vi "Measurement UI.vi"() -> ()   [LabVIEW 2022 SP3, in "Frequency Response UI.lvlib"]
uses:
  Frequency Response UI.lvlib
  shared/controls/sweep profile.ctl
  shared/ui/controls/view.ctl
  shared/controls/input type.ctl
  UI State.ctl
  <vilib>/Utility/miscctls.llb/LVBoundsTypeDef.ctl
  <vilib>/Utility/miscctls.llb/LVPoint32TypeDef.ctl
  <vilib>/Utility/miscctls.llb/LVPointTypeDef.ctl
  Y axis data selection.ctl
  shared/ui/UI Helpers.lvlib
  shared/configuration dialogs/Config Dialog.lvlib
  shared/input configuration file/input cfg file.lvlib
panel:
  in  "view legend":T1
  out "plot point":string
  out "Sweep graph":cluster{"frequency (Hz)":dbl[], "THD+N":dbl[]}[](graph)
  out "Time domain graph":waveform(dbl)[](graph)
  in  "y-axis mapping":enum32{"linear", "logarithmic"}(ring) caption="Y-axis mapping"
  in  "output channel":string="PXI1Slot4/ai0"
  out "ref mic wfm - data":dbl[](array[numeric])
  out "ref mic wfm - dt":dbl
  in  "input cfg file":string
  out "THD":dbl[](array[numeric])
  out "THD+N":dbl[](array[numeric])
  out "amplitude (dBr)":dbl[](array[numeric])
  out "frequency (Hz)":dbl[](array[numeric])
  in  "Configuration tab":T2(tab)
  in  "digital mic sensitivity (dBFS)":dbl=-26.0 caption="Microphone Sensitivity" format="%#.6p dBFS"
  in  "input type":T3 caption="Input Type"
  out "input cfg file name":string
  in  "configure input":bool
  in  "digital channel list":string caption="Digital Audio Channel"
  in  "Output Channel":tag="PXI1Slot2/ao0" caption="Channel"
  in  "Ref Mic Channel":tag="PXI1Slot2/ai0" caption="Channel"
  in  "ref mic sensitivity (mV/Pa)":dbl=50.0 caption="Sensitivity" format="%#.6f mV/Pa"
  in  "output level (dBSPL)":dbl=94.0 caption="Output level" format="%#_3f dBSPL"
  in  "output voltage ratio":dbl=3.39 caption="Output voltage ratio" format="%.3p Pa/V"
  in  "min settling cycles":u32 caption="Minimum settling cycles"
  in  "min settling time (s)":dbl=0.1 caption="Minimum settling time" format="%#_6ps"
  in  "sweep profile":T4=enum."Logarithmic" caption="Profile"
  in  "number of steps":dbl=20000.0 caption="Number of steps"
  in  "start frequency":dbl=20.0 caption="Sweep start" format="%#_6pHz"
  in  "stop frequency":dbl=20000.0 caption="Sweep stop" format="%#_6pHz"
  in  "min measurement cycles":u32 caption="Minimum measurement cycles"
  in  "min measurement time (s)":dbl=0.1 caption="Minimum measurement time" format="%#_6ps"
  in  "x-axis mapping":enum32{"linear", "logarithmic"}(ring) caption="X-axis mapping"
  out "wfm - data":dbl[](array[numeric])
  out "wfm - dt":dbl
  out "channel name":string
  in  "ref mic channel":string="PXI1Slot4/ai0"
  # "hidden controls - used to sync with MeasLink"
  # "hidden for future use"
  # "hidden indicators"
  # "Microphone Interface"
  # "Harware Resource"
  # "Output"
  # "Reference Microphone"
  # "Measurement Settings"
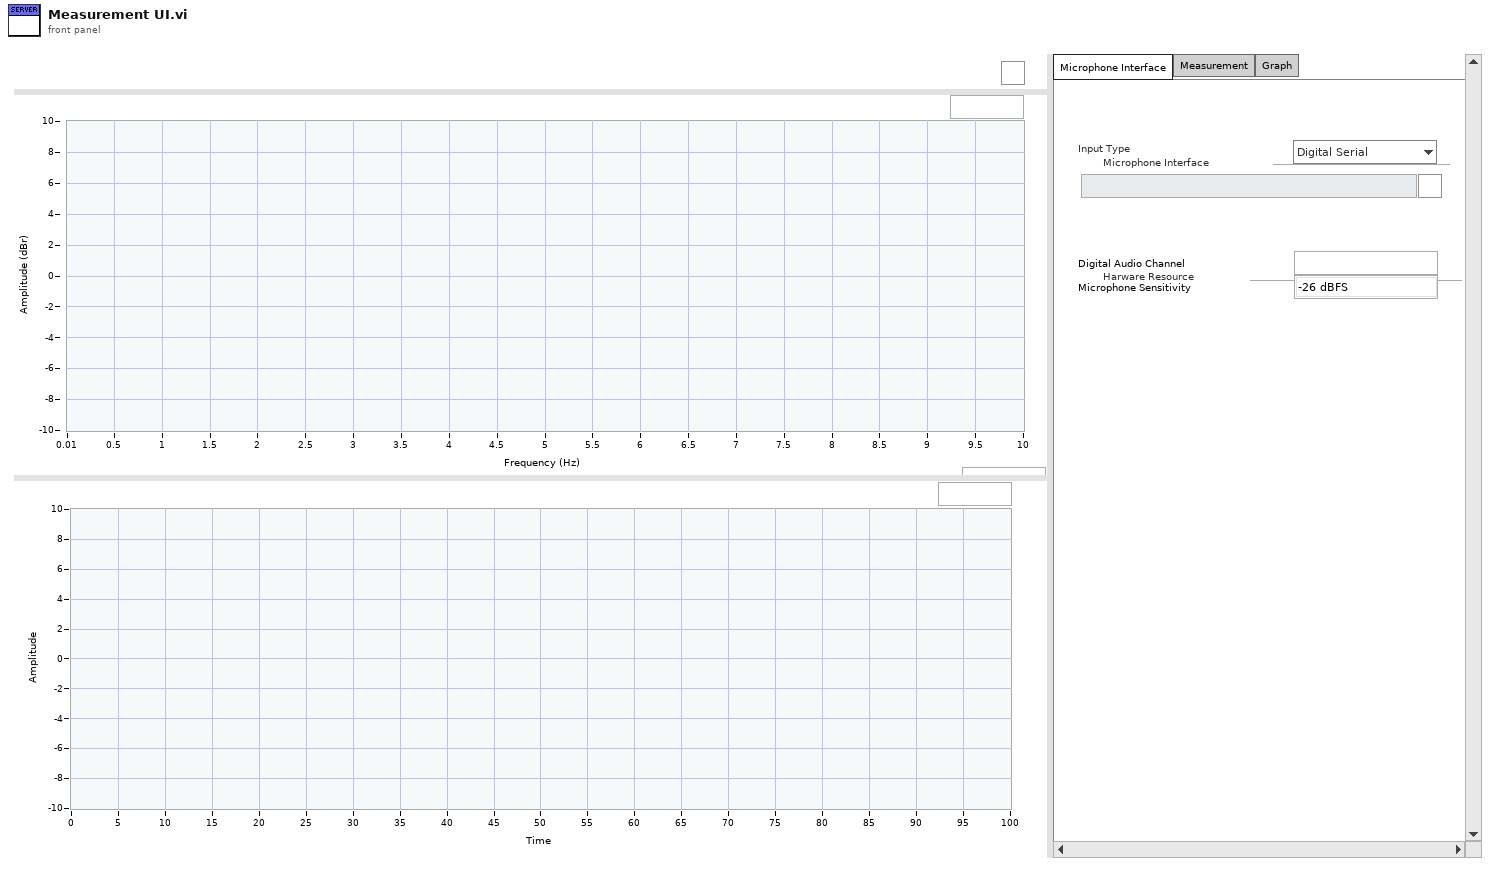
[diagram p1: front panel]
types:
  T1 = typedef "UI Helpers.lvlib/view.ctl" = bool
  T2 = enum32{"Microphone Interface", "Measurement", "Graph"}
  T3 = typedef "input type.ctl" = enum32{"Digital Serial", "PDM"}
  T4 = typedef "sweep profile.ctl" = enum32{"Linear", "Logarithmic"}
  T5 = typedef "Frequency Response UI.lvlib/UI State.ctl" = cluster{"Graph Size":T6, "Legend Visible":bool, "Mouse Coords":T7, "Visible Plot Id":i32, "PostUI event occurred":bool, "input cfg file":path}
  T6 = typedef "LVBoundsTypeDef.ctl" = cluster{"Width":u32, "Height":u32}
  T7 = typedef "LVPoint32TypeDef.ctl" = cluster{"Horizontal":i32, "Vertical":i32}
  T8 = typedef "Frequency Response UI.lvlib/Y axis data selection.ctl" = enum32{"Amplitude (dBr)", "THD (%)", "THD+N (%)"}
  T9 = typedef "LVPointTypeDef.ctl" = cluster{"Horizontal":i16, "Vertical":i16}
  T10 = typedef "Config Dialog.lvlib/audio settings.ctl" = cluster{"input cfg file":string}
  T11 = cluster{"frequency (Hz)":dbl[], "amplitude (dBr)":dbl[]}
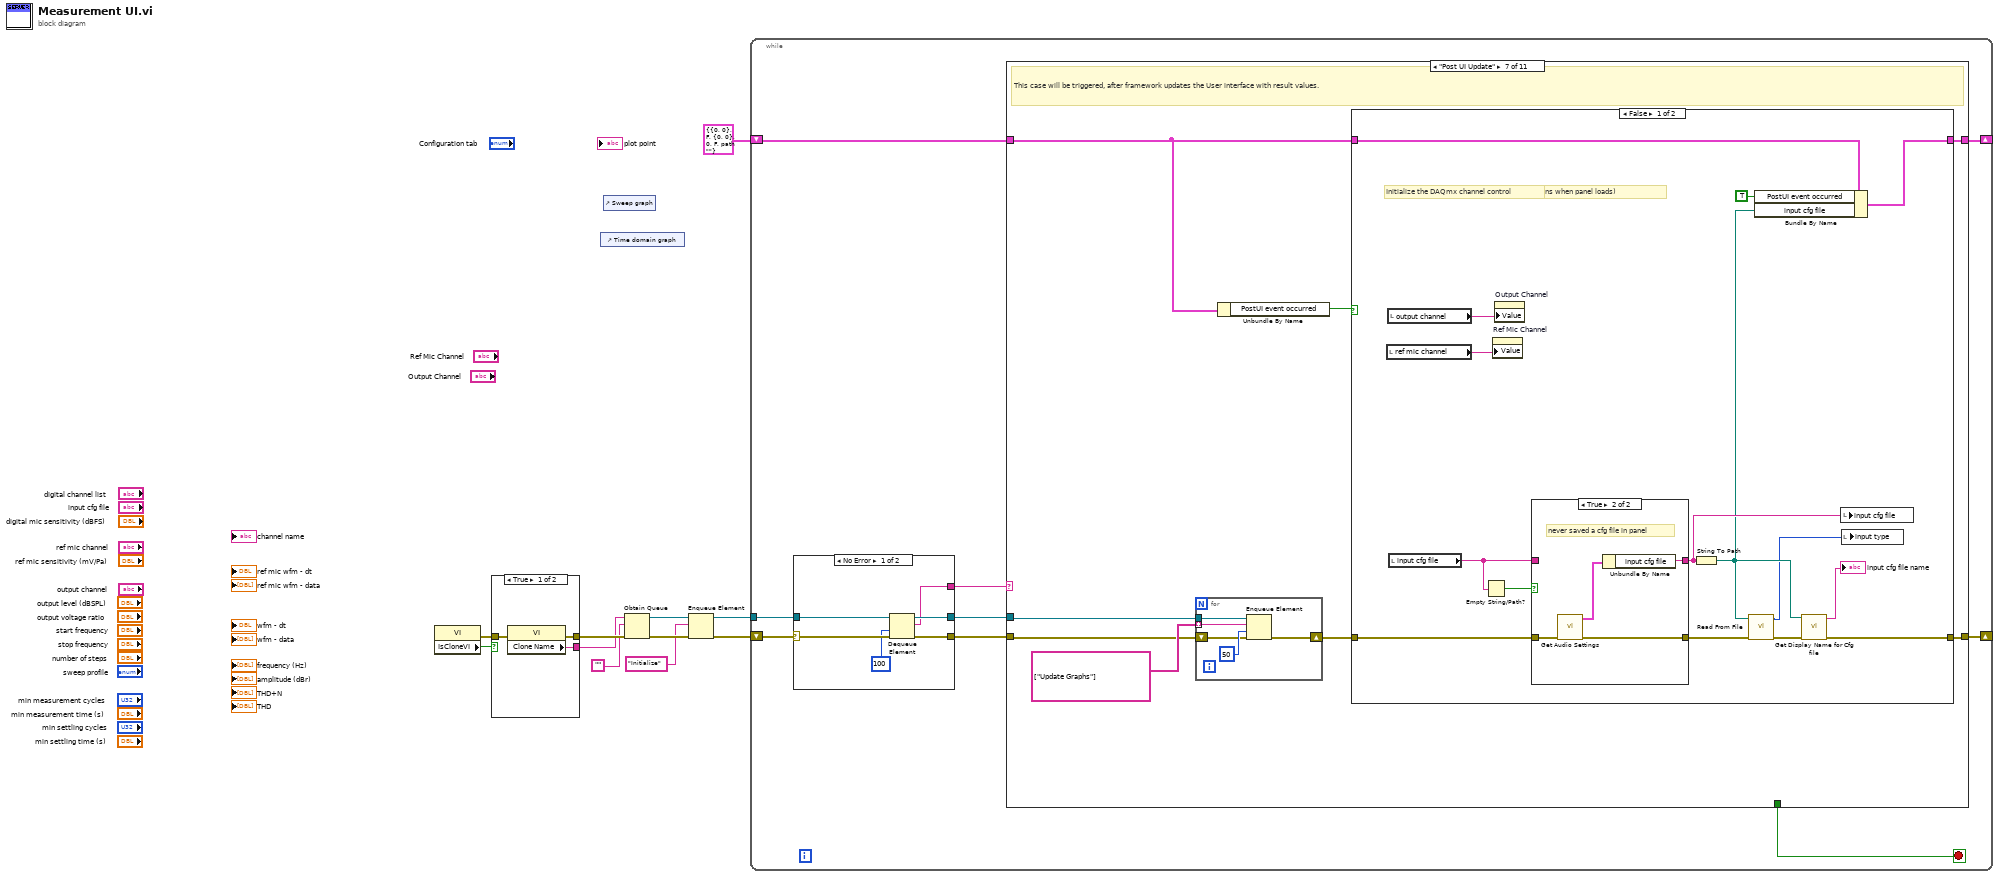
[diagram p0: block diagram]
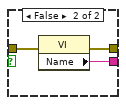
[diagram p2: hidden frame]
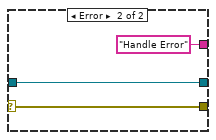
[diagram p3: hidden frame]
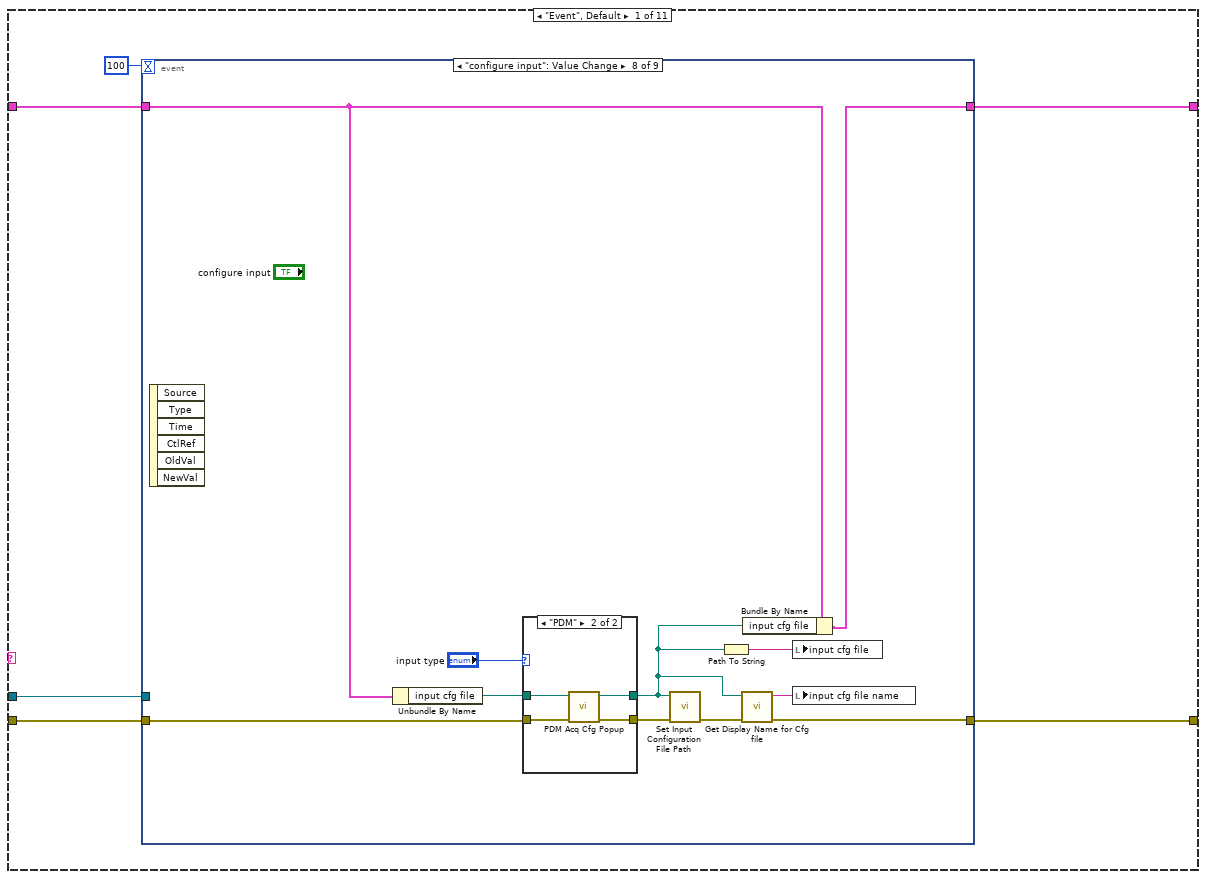
[diagram p4: hidden frame]
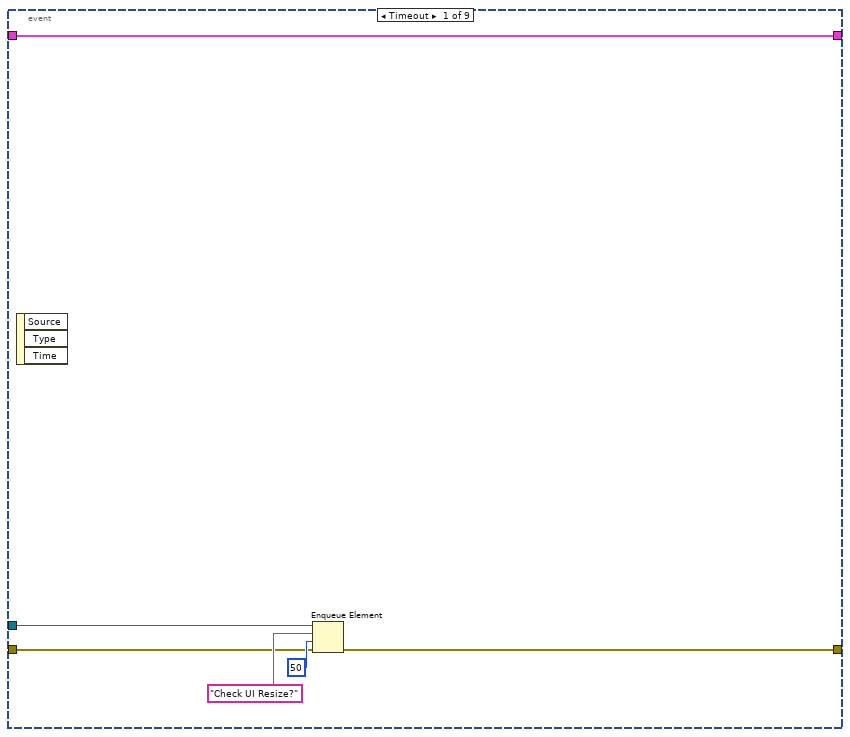
[diagram p5: hidden frame]
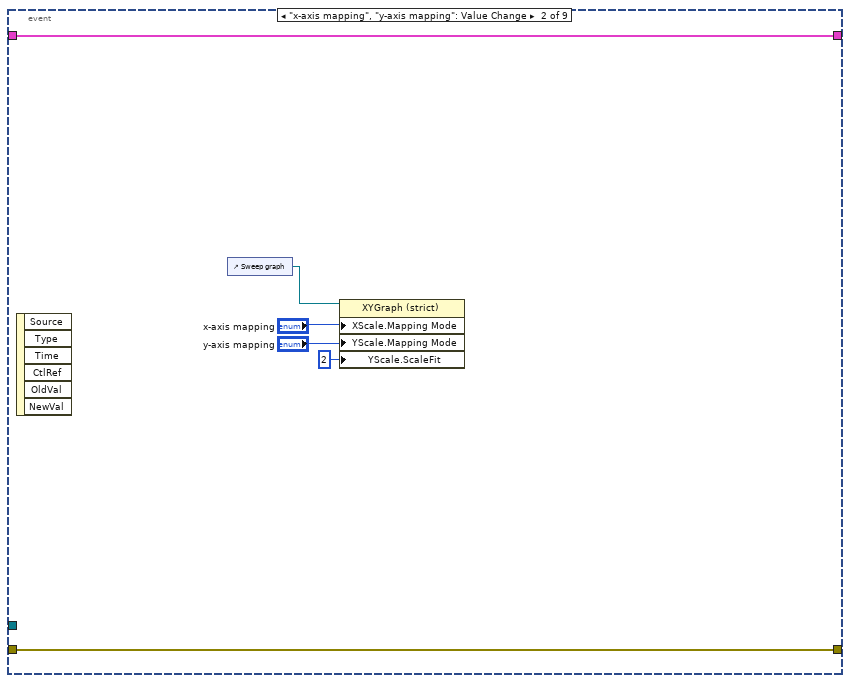
[diagram p6: hidden frame]
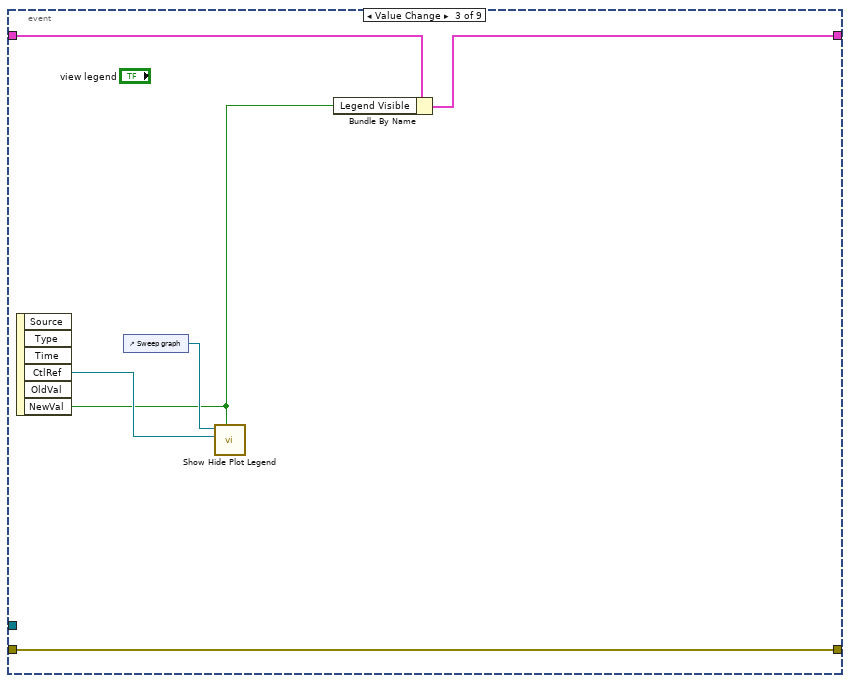
[diagram p7: hidden frame]
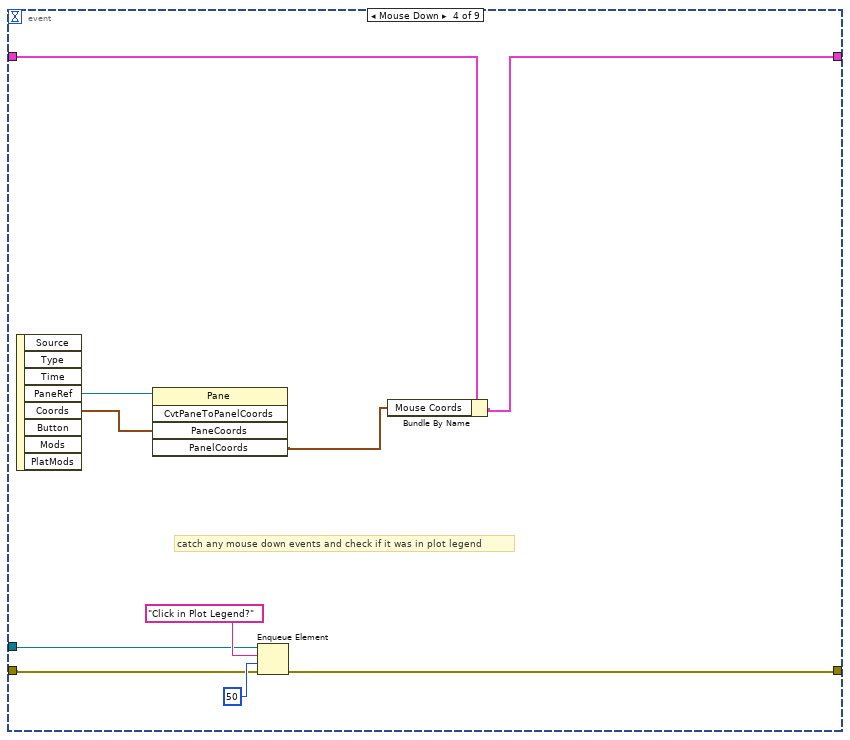
[diagram p8: hidden frame]
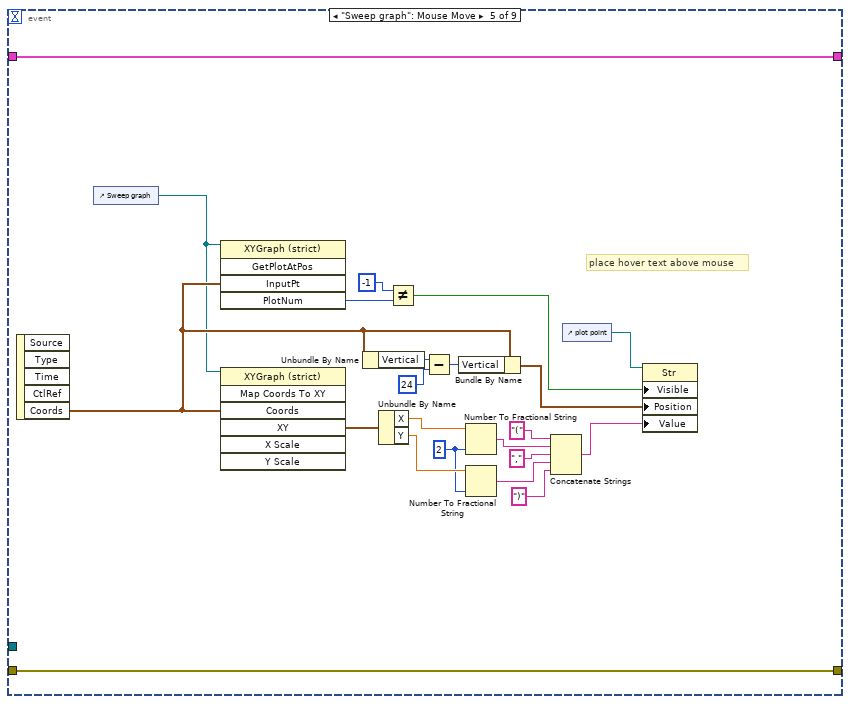
[diagram p9: hidden frame]
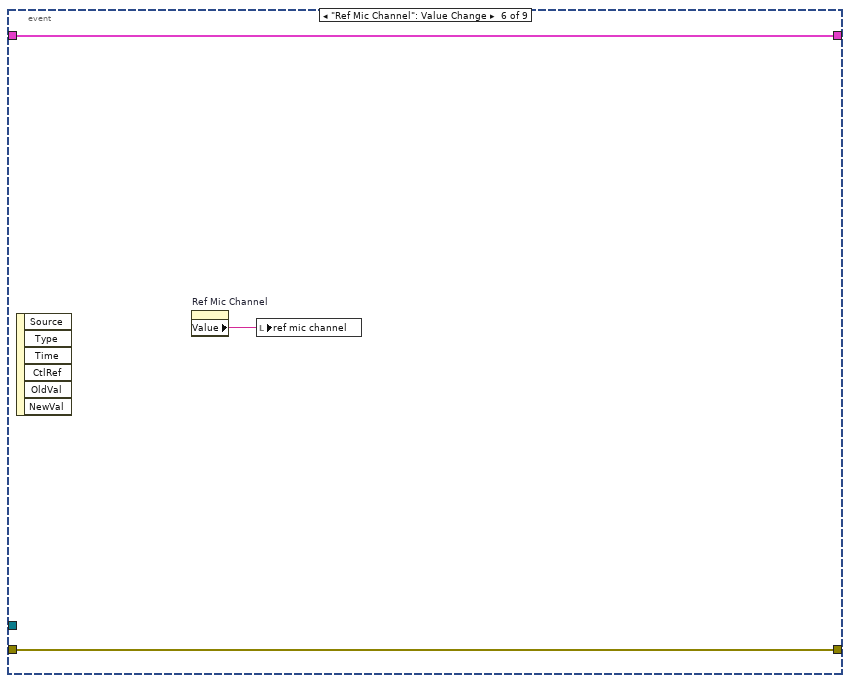
[diagram p10: hidden frame]
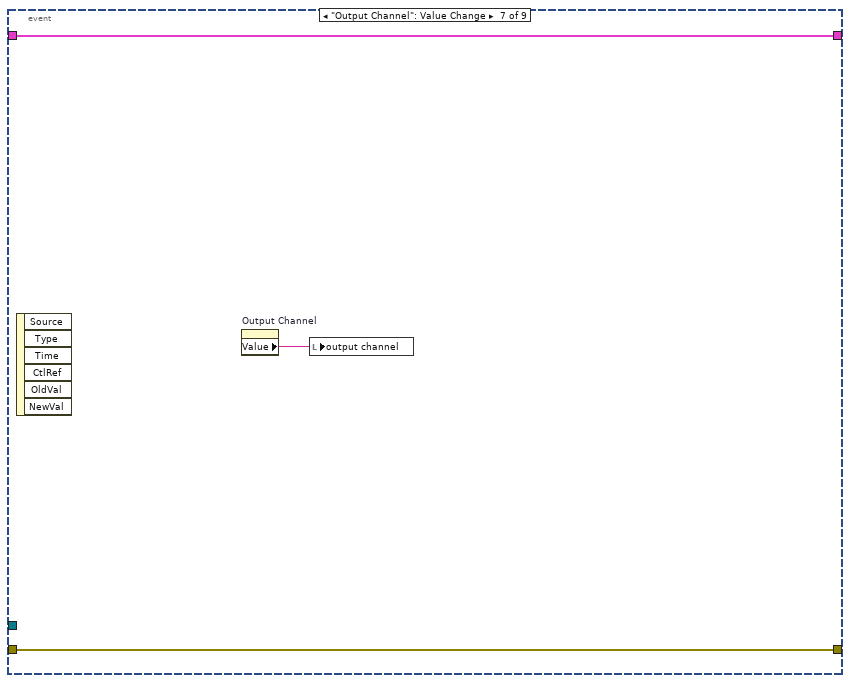
[diagram p11: hidden frame]
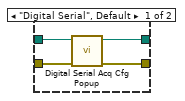
[diagram p12: hidden frame]
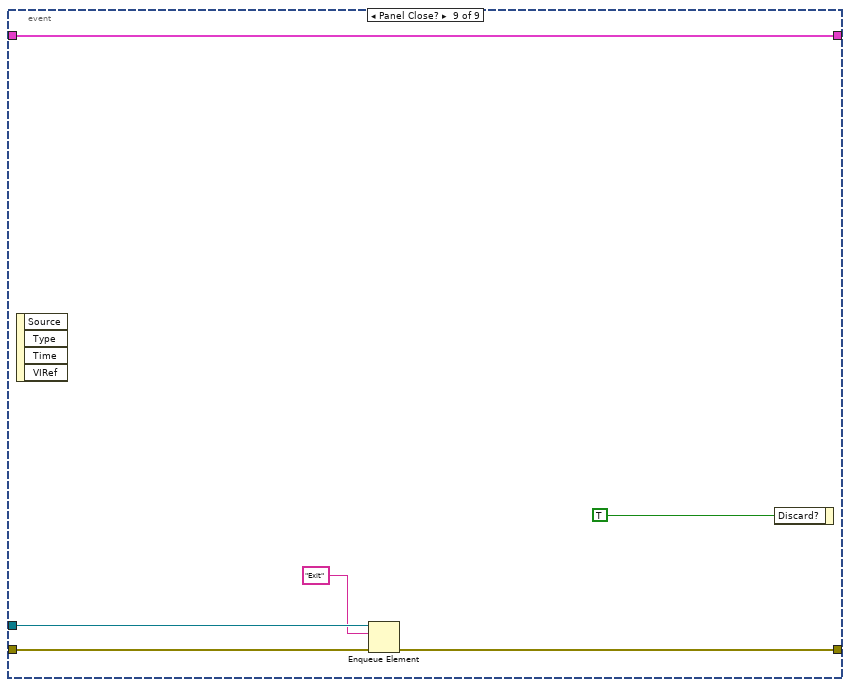
[diagram p13: hidden frame]
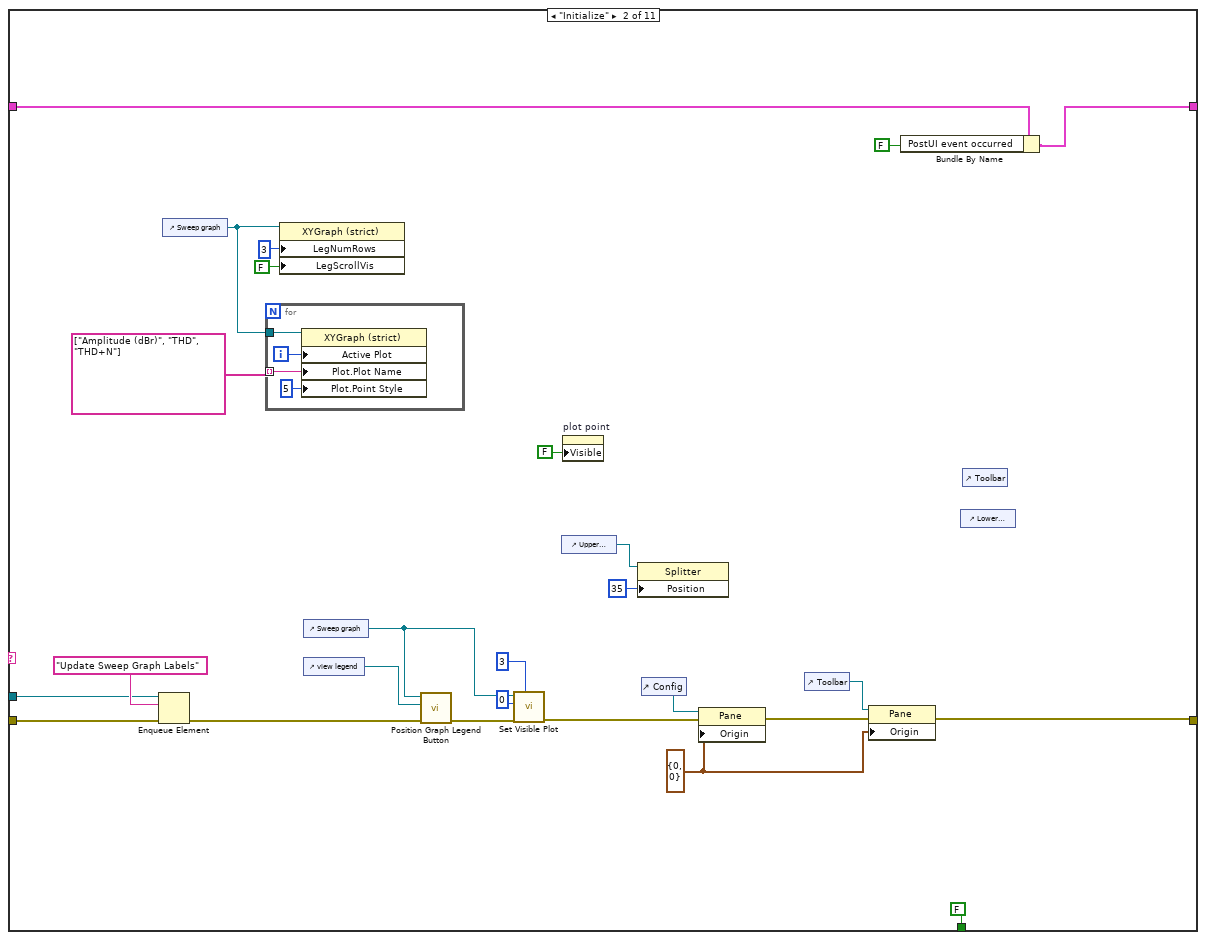
[diagram p14: hidden frame]
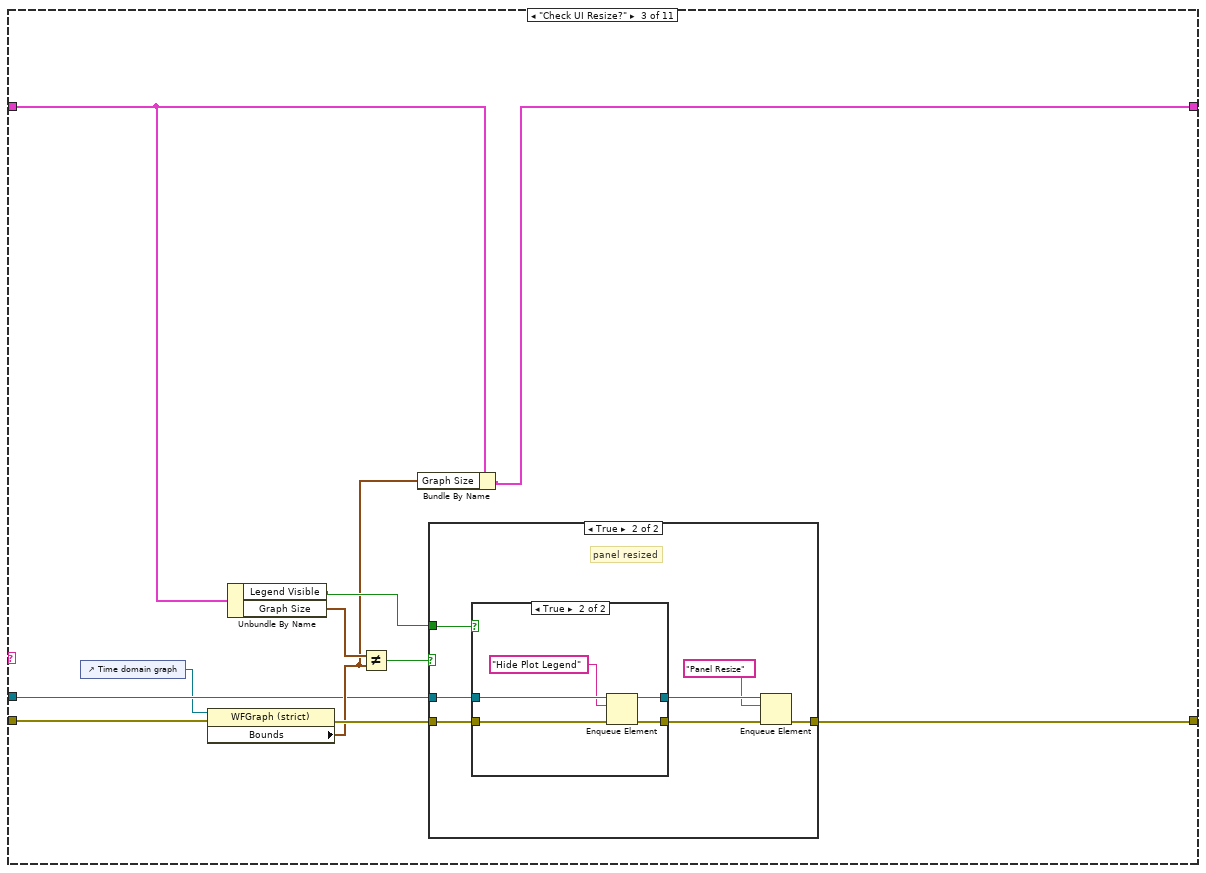
[diagram p15: hidden frame]
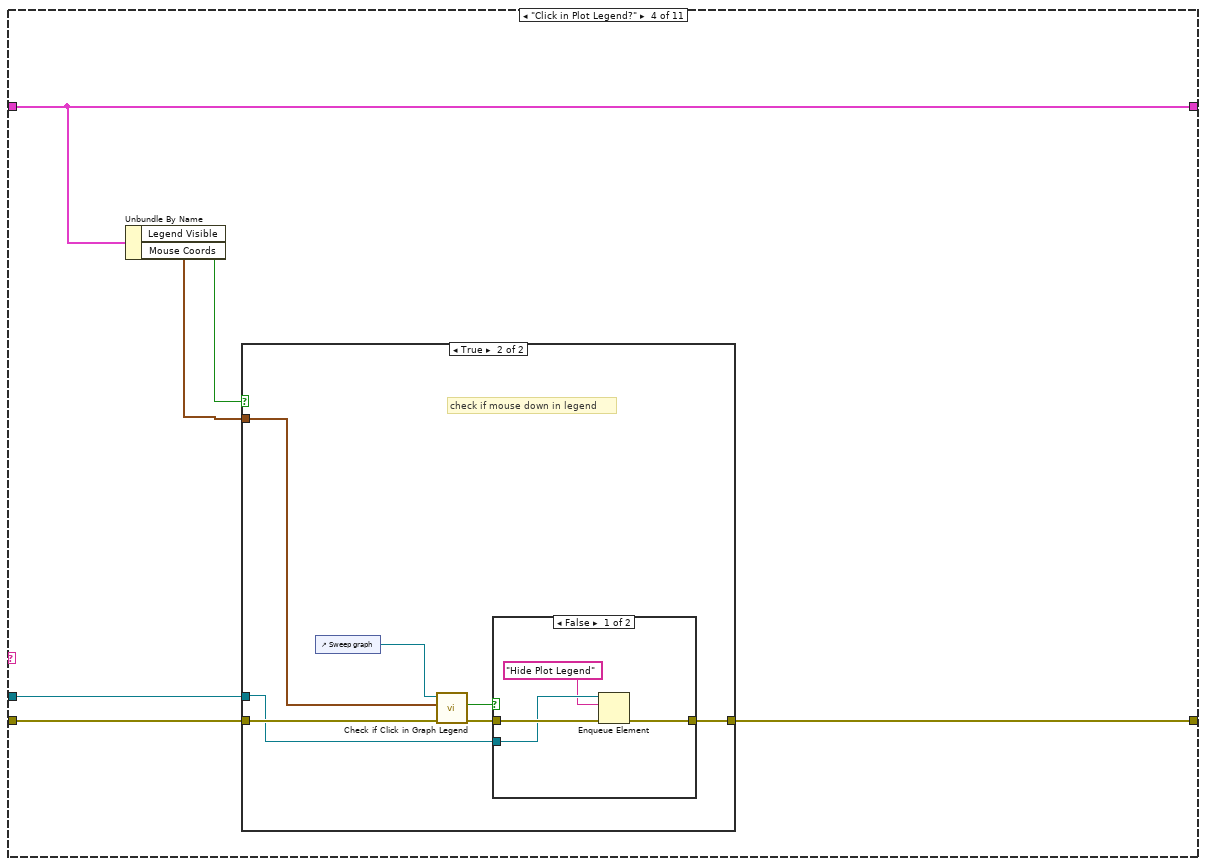
[diagram p18: hidden frame]
diagram:
  n1 = property class="VI"() -> (error out=w2:errorcluster, "IsCloneVI"=w3:bool)  [unwired: 2 in, 1 out]
  n2 = case shown="True" w3 {
    tunnel: [w14 w17] -> w11
    tunnel: [w13 w16] -> w10
    tunnel: w2 -> [w12 w15]
    frame True {
      n3 = property class="VI"(error in=w12) -> (error out=w14:errorcluster, "Clone Name"=w13:string)  [unwired: 1 in, 1 out]
    }
    frame False {
      n4 = property class="VI"(error in=w15) -> (error out=w17:errorcluster, "Name"=w16:string)  [unwired: 1 in, 1 out]
    }
  }
  n5 = control-ref of="Time domain graph"() -> ()  [unwired: 1 out]
  n6 = control-ref of="Sweep graph"() -> ()  [unwired: 1 out]
  n7 = Obtain Queue(name (unnamed)=w10, element data type="", error in (no error)=w11) -> (queue out=w7:refnum<queue>, error out=w9:errorcluster)  [unwired: 2 in, 1 out]
  n8 = Enqueue Element(queue=w7, element="Initialize", error in (no error)=w9) -> (queue out=w6:refnum<queue>, error out=w8:errorcluster)  [unwired: 1 in, 1 out]
  n9 = while {
    shift-right: [w21] -> _
    shift-left: w8 -> [w26]
    tunnel: w6 -> [w24]
    shift-right: [w18] -> _
    shift-left: T5 {"Graph Size"={"Width"=0, "Height"=0}, "Legend Visible"=FALSE, "Mouse Coords"={"Horizontal"=0, "Vertical"=0}, "Visible Plot Id"=0, "PostUI event occurred"=FALSE, "input cfg file"=path ""} ("UI State") -> [w19]
    stop <- w20 stop-if-true
    n10 = case shown="No Error" w26 {
      selector: w26 -> [w32 w35]
      tunnel: [w31 w35] -> w25
      tunnel: w24 -> [w30 w34]
      tunnel: [w29 w34] -> w23
      tunnel: [w28 "Handle Error"] -> w22
      frame No Error {
        n11 = Dequeue Element(queue=w30, timeout in ms (-1)=100, error in (no error)=w32) -> (queue out=w29:refnum<queue>, element=w28:string, error out=w31:errorcluster)  [unwired: 1 out]
      }
      frame Error {
      }
    }
    n12 = case shown="\"Post UI Update\"" w22 {
      tunnel: w25 -> [w40 w139 w157 w182 w202 w207 w216 w262 w271 w279 w281]
      tunnel: w23 -> [w38 w138 w158 w181 _ _ w217 _ _ w277 _]
      tunnel: [w41 w124 w156 w179 w201 w206 w214 w262 w271 w274 w281] -> w21
      tunnel: [_ FALSE _ _ _ _ _ _ _ TRUE _] -> w20
      tunnel: w19 -> [w37 w129 w155 w180 w204 w210 w211 w263 w270 w272 w280]
      tunnel: [w36 w128 w154 w180 w203 w210 w213 w263 w270 w272 w280] -> w18
      frame "Event", Default {
        n13 = event shown="[7] \"configure input\": Value Change" {
          selector: _ -> [_ _ _ _ _ _ _ _ _]
          dyn-events: _ -> [_ _ _ _ _ _ _ _ _]
          timeout: 100 -> [_ _ _ _ _ _ _ _ _]
          tunnel: [w45 w49 w54 w60 w91 w94 w97 w101 w120] -> w41
          tunnel: w40 -> [w44 w49 w54 w61 w91 w94 w97 w102 w121]
          tunnel: w38 -> [w43 _ _ w62 _ _ _ _ w119]
          tunnel: w37 -> [w42 w48 w56 w66 w90 w93 w96 w104 w117]
          tunnel: [w42 w48 w55 w65 w90 w93 w96 w103 w117] -> w36
          event Timeout {
            n14 = event-data() -> ()  [unwired: 1 in, 3 out]
            n15 = Enqueue Element(queue=w43, element="Check UI Resize?", timeout in ms (-1)=50, error in (no error)=w44) -> (error out=w45:errorcluster)  [unwired: 2 out]
          }
          event "x-axis mapping", "y-axis mapping": Value Change {
            n16 = event-data() -> ()  [unwired: 1 in, 6 out]
            n17 = control-ref of="Sweep graph"() -> (w50:refnum<vi>)
            n18 = property on="Property Node" class="XYGraph (strict)"(reference=w50, "XScale.Mapping Mode"="x-axis mapping", "YScale.Mapping Mode"="y-axis mapping", "YScale.ScaleFit"=u8 2 ("Y Scale.Scale Fit")) -> ()  [unwired: 1 in, 2 out]
          }
          event Value Change {
            n19 = event-data() -> ("CtlRef"=w59:refnum<vi>, "NewVal"=w57:T1)  [unwired: 1 in, 4 out]
            n20 = control-ref of="Sweep graph"() -> (w58:refnum<vi>)
            n21 = call "Show Hide Plot Legend.vi"("show"=w57, "view reference"=w59, "graph reference"=w58) -> ()  [unwired: 8 in, 1 out]
            n22 = Bundle By Name(cluster=w56, "Legend Visible"=w57) -> (w55:T5)
          }
          event Mouse Down {
            # "catch any mouse down events and check if it was in plot legend"
            n23 = event-data() -> ("PaneRef"=w68:refnum<vi>, "Coords"=w67:T7)  [unwired: 1 in, 6 out]
            n24 = invoke class="Pane" method="CvtPaneToPanelCoords"(reference=w68, "PaneCoords"=w67) -> ("PanelCoords"=w69:T9)  [unwired: 3 in, 4 out]
            n25 = Enqueue Element(queue=w62, element="Click in Plot Legend?", timeout in ms (-1)=50, error in (no error)=w61) -> (error out=w60:errorcluster)  [unwired: 2 out]
            n26 = Bundle By Name(cluster=w66, "Mouse Coords"=w69) -> (w65:T5)
          }
          event "Sweep graph": Mouse Move {
            w73 = i16 2 ("precision (6)")
            # "place hover text above mouse"
            n27 = event-data() -> ("Coords"=w71:T7)  [unwired: 1 in, 4 out]
            n28 = control-ref of="Sweep graph"() -> (w70:refnum<vi>)
            n29 = invoke class="XYGraph (strict)" method="GetPlotAtPos"(reference=w70, "InputPt"=w71) -> ("PlotNum"=w79:i32)  [unwired: 3 in, 4 out]
            n30 = invoke class="XYGraph (strict)" method="Map Coords To XY"(reference=w70, "Coords"=w71) -> ("XY"=w78:cluster{"X":dbl, "Y":dbl})  [unwired: 5 in, 6 out]
            n31 = Unbundle By Name(w71) -> ("Vertical"=w87:i32)
            n32 = Unbundle By Name(w78) -> ("X"=w84:dbl, "Y"=w85:dbl)
            n33 = Not Equal?(x=-1, y=w79) -> (x != y?=w80:bool)
            n34 = Subtract(x=w87, y=24) -> (x-y=w88:i32)
            n35 = Bundle By Name(cluster=w71, "Vertical"=w88) -> (w86:T7)
            n36 = Number To Fractional String(number=w84, precision (6)=w73) -> (F-format string=w81:string)  [unwired: 2 in]
            n37 = Number To Fractional String(number=w85, precision (6)=w73) -> (F-format string=w82:string)  [unwired: 2 in]
            n38 = Concatenate Strings("(" ("string"), w81, "," ("string"), w82, ")" ("string")) -> (w83:string)
            n39 = control-ref of="plot point"() -> (w89:refnum<vi>)
            n40 = property on="Property Node" class="Str"(reference=w89, "Visible"=w80, "Position"=w86, "Value"=w83) -> ()  [unwired: 1 in, 2 out]
          }
          event "Ref Mic Channel": Value Change {
            n41 = event-data() -> ()  [unwired: 1 in, 6 out]
            n42 = property on="Ref Mic Channel" class="DAQmxName"() -> ("Value"=w92:string)  [unwired: 2 in, 2 out]
            n43 = local write "ref mic channel"(w92) -> ()
          }
          event "Output Channel": Value Change {
            n44 = event-data() -> ()  [unwired: 1 in, 6 out]
            n45 = property on="Output Channel" class="DAQmxName"() -> ("Value"=w95:string)  [unwired: 2 in, 2 out]
            n46 = local write "output channel"(w95) -> ()
          }
          event "configure input": Value Change {
            n47 = event-data() -> ()  [unwired: 1 in, 6 out]
            n48 = Unbundle By Name(w104) -> ("input cfg file"=w108:path)
            n49 = case shown="\"PDM\"" "input type" {
              tunnel: w108 -> [w112 w116]
              tunnel: w102 -> [w111 w115]
              tunnel: [w110 w113] -> w107
              tunnel: [w109 w114] -> w105
              frame "Digital Serial", Default {
                n50 = call "Digital Serial Acq Cfg Popup.vi"("error in (no error)"=w111, "config file in"=w112) -> ("error out"=w110:errorcluster, "config file out"=w109:path)  [unwired: 7 in, 1 out]
              }
              frame "PDM" {
                n51 = call "PDM Acq Cfg Popup.vi"("error in (no error)"=w115, "config file in"=w116) -> ("error out"=w113:errorcluster, "config file out"=w114:path)  [unwired: 7 in, 1 out]
              }
            }
            n52 = call "Set Input Configuration File Path.vi"("error in (no error)"=w107, "configuration file"=w105) -> ("error out"=w106:errorcluster)  [unwired: 9 in]
            n53 = Path To String(path=w105) -> (string=w99:string)
            n54 = call "Get Display Name for Cfg file.vi"("error in (no error)"=w106, "file path"=w105) -> ("error out"=w101:errorcluster, "display string"=w98:string)  [unwired: 8 in]
            n55 = Bundle By Name(cluster=w104, "input cfg file"=w105) -> (w103:T5)
            n56 = local write "input cfg file"(w99) -> ()
            n57 = local write "input cfg file name"(w98) -> ()
          }
          event Panel Close? {
            n58 = event-data() -> ()  [unwired: 1 in, 4 out]
            n59 = Enqueue Element(queue=w119, element="Exit", error in (no error)=w121) -> (error out=w120:errorcluster)  [unwired: 1 in, 2 out]
            n60 = event-data("Discard?"=TRUE) -> ()  [unwired: 1 in, 1 out]
          }
        }
      }
      frame "Initialize" {
        w125 = T9 {"Horizontal"=0, "Vertical"=0} ("Origin")
        n61 = Enqueue Element(queue=w138, element="Update Sweep Graph Labels", error in (no error)=w139) -> (error out=w136:errorcluster)  [unwired: 1 in, 2 out]
        n62 = control-ref of="Sweep graph"() -> (w141:refnum<vi>)
        n63 = for {
          tunnel: string[] ["Amplitude (dBr)", "THD", "THD+N"] -> [w151] mode=indexing
          tunnel: w141 -> [w150]
          i -> [w152]
          n64 = property on="Property Node" class="XYGraph (strict)"(reference=w150, "Active Plot"=w152, "Plot.Plot Name"=w151, "Plot.Point Style"=u8 5) -> ()  [unwired: 1 in, 2 out]
        }
        n65 = property class="XYGraph (strict)"(reference=w141, "LegNumRows"=u32 3 ("Legend:Number of Rows"), "LegScrollVis"=FALSE ("Legend:Scrollbar Visible")) -> ()  [unwired: 1 in, 2 out]
        n66 = control-ref of="Sweep graph"() -> (w135:refnum<vi>)
        n67 = control-ref of="view legend"() -> (w137:refnum<vi>)
        n68 = call "Position Graph Legend Button.vi"("error in (no error)"=w136, "view legend"=w137, "graph"=w135) -> ("error out"=w133:errorcluster)  [unwired: 8 in]
        n69 = call "Set Visible Plot.vi"("number of plots"=3, "error in (no error)"=w133, "Plot Id"=0, "XYGraph in"=w135) -> ("error out"=w132:errorcluster)  [unwired: 7 in]
        n70 = control-ref of="Upper Splitter"() -> (w146:refnum<vi>)
        n71 = property on="plot point" class="Str"("Visible"=FALSE) -> ()  [unwired: 2 in, 2 out]
        n72 = property class="Splitter"(reference=w146, "Position"=35 ("Position:Top")) -> ()  [unwired: 1 in, 2 out]
        n73 = control-ref of="Config"() -> (w147:refnum<vi>)
        n74 = property class="Pane"(reference=w147, error in=w132, "Origin"=w125) -> (error out=w126:errorcluster)  [unwired: 1 out]
        n75 = control-ref of="Toolbar"() -> (w123:refnum<vi>)
        n76 = property class="Pane"(reference=w123, error in=w126, "Origin"=w125) -> (error out=w124:errorcluster)  [unwired: 1 out]
        n77 = Bundle By Name(cluster=w129, "PostUI event occurred"=FALSE) -> (w128:T5)
        n78 = control-ref of="Lower Splitter"() -> ()  [unwired: 1 out]
        n79 = control-ref of="Toolbar"() -> ()  [unwired: 1 out]
      }
      frame "Check UI Resize?" {
        n80 = control-ref of="Time domain graph"() -> (w153:refnum<vi>)
        n81 = property on="Property Node" class="WFGraph (strict)"(reference=w153, error in=w157) -> (error out=w163:errorcluster, "Bounds"=w159:T6)  [unwired: 1 out]
        n82 = Unbundle By Name(w155) -> ("Legend Visible"=w161:bool, "Graph Size"=w160:T6)
        n83 = Not Equal?(x=w160, y=w159) -> (x != y?=w162:bool)
        n84 = Bundle By Name(cluster=w155, "Graph Size"=w159) -> (w154:T5)
        n85 = case shown="True" w162 {
          tunnel: w163 -> [w164 w171]
          tunnel: [w164 w166] -> w156
          tunnel: w161 -> [_ w169]
          tunnel: w158 -> [_ w170]
          frame False {
            # "no resize"
          }
          frame True {
            # "panel resized"
            n86 = case shown="True" w169 {
              tunnel: w171 -> [w173 w178]
              tunnel: [w173 w177] -> w168
              tunnel: w170 -> [w172 w176]
              tunnel: [w172 w174] -> w167
              frame False {
              }
              frame True {
                n87 = Enqueue Element(queue=w176, element="Hide Plot Legend", error in (no error)=w178) -> (queue out=w174:refnum<queue>, error out=w177:errorcluster)  [unwired: 1 in, 1 out]
              }
            }
            n88 = Enqueue Element(queue=w167, element="Panel Resize", error in (no error)=w168) -> (error out=w166:errorcluster)  [unwired: 1 in, 2 out]
          }
        }
      }
      frame "Click in Plot Legend?" {
        n89 = Unbundle By Name(w180) -> ("Legend Visible"=w183:bool, "Mouse Coords"=w184:T7)
        n90 = case shown="True" w183 {
          tunnel: w184 -> [_ w191]
          tunnel: w181 -> [_ w188]
          tunnel: w182 -> [w185 w192]
          tunnel: [w185 w187] -> w179
          frame False {
            # "legend not visible; do nothing"
          }
          frame True {
            # "check if mouse down in legend"
            n91 = control-ref of="Sweep graph"() -> (w186:refnum<vi>)
            n92 = call "Check if Click in Graph Legend.vi"("error in (no error)"=w192, "Mouse Coords"=w191, "WaveformGraph"=w186) -> ("error out"=w189:errorcluster, "click in legend?"=w190:bool)  [unwired: 7 in]
            n93 = case shown="False" w190 {
              tunnel: w189 -> [w196 w197]
              tunnel: w188 -> [w195 _]
              tunnel: [w194 w197] -> w187
              frame False {
                n94 = Enqueue Element(queue=w195, element="Hide Plot Legend", error in (no error)=w196) -> (error out=w194:errorcluster)  [unwired: 1 in, 2 out]
              }
              frame True {
                # "inside legend; do nothing"
              }
            }
          }
        }
      }
      frame "Hide Plot Legend" {
        n95 = control-ref of="Sweep graph"() -> (w199:refnum<vi>)
        n96 = control-ref of="view legend"() -> (w200:refnum<vi>)
        n97 = Bundle By Name(cluster=w204, "Legend Visible"=FALSE ("legend visible")) -> (w203:T5)
        n98 = call "Show Hide Plot Legend.vi"("show"=FALSE, "error in (no error)"=w202, "view reference"=w200, "graph reference"=w199) -> ("error out"=w201:errorcluster)  [unwired: 7 in]
      }
      frame "Panel Resize" {
        n99 = control-ref of="Sweep graph"() -> (w208:refnum<vi>)
        n100 = control-ref of="view legend"() -> (w209:refnum<vi>)
        n101 = call "Position Graph Legend Button.vi"("error in (no error)"=w207, "view legend"=w209, "graph"=w208) -> ("error out"=w206:errorcluster)  [unwired: 8 in]
      }
      frame "Post UI Update" {
        # "This case will be triggered, after framework updates the User interface with result values."
        n102 = for {
          tunnel: w217 -> [w244]
          shift-right: [w243] -> w215
          shift-left: w216 -> [w245]
          tunnel: string[] ["Update Graphs"] -> [w242] mode=indexing
          n103 = Enqueue Element(queue=w244, element=w242, timeout in ms (-1)=50, error in (no error)=w245) -> (error out=w243:errorcluster)  [unwired: 2 out]
        }
        n104 = Unbundle By Name(w211) -> ("PostUI event occurred"=w212:bool)
        n105 = case shown="False" w212 {
          tunnel: w215 -> [w228 w241]
          tunnel: [w222 w241] -> w214
          tunnel: w211 -> [w231 w240]
          tunnel: [w230 w240] -> w213
          frame False {
            # "do this on first PostUI Event (happens when panel loads)"
            # "Initialize the DAQmx channel control"
            n106 = local read "ref mic channel"() -> (w233:string)
            n107 = local read "output channel"() -> (w225:string)
            n108 = local read "input cfg file"() -> (w227:string)
            n109 = Empty String/Path?(string/path=w227) -> (empty?=w229:bool)
            n110 = property on="Ref Mic Channel" class="DAQmxName"("Value"=w233) -> ()  [unwired: 2 in, 2 out]
            n111 = property on="Output Channel" class="DAQmxName"("Value"=w225) -> ()  [unwired: 2 in, 2 out]
            n112 = case shown="True" w229 {
              tunnel: w228 -> [w235 w239]
              tunnel: [w235 w237] -> w223
              tunnel: w227 -> [w234 _]
              tunnel: [w234 w236] -> w226
              frame False {
              }
              frame True {
                # "never saved a cfg file in panel"
                n113 = call "Get Audio Settings.vi"("error in (no error)"=w239) -> ("error out"=w237:errorcluster, "audio settings"=w238:T10)  [unwired: 9 in]
                n114 = Unbundle By Name(w238) -> ("input cfg file"=w236:string)
              }
            }
            n115 = String To Path(string=w226) -> (path=w220:path)
            n116 = call "Read From File.vi"("error in (no error)"=w223, "file path"=w220) -> ("error out"=w224:errorcluster, "input type"=w219:T3)  [unwired: 6 in, 2 out]
            n117 = Bundle By Name(cluster=w231, "PostUI event occurred"=TRUE, "input cfg file"=w220) -> (w230:T5)
            n118 = call "Get Display Name for Cfg file.vi"("error in (no error)"=w224, "file path"=w220) -> ("error out"=w222:errorcluster, "display string"=→"input cfg file name":string)  [unwired: 8 in]
            n119 = local write "input cfg file"(w226) -> ()
            n120 = local write "input type"(w219) -> ()
          }
          frame True {
          }
        }
      }
      frame "Update Graphs" {
        n121 = local read "amplitude (dBr)"() -> (w253:dbl[])
        n122 = local read "frequency (Hz)"() -> (w254:dbl[])
        n123 = local read "ref mic wfm - data"() -> (w257:dbl[])
        n124 = local read "THD+N"() -> (w251:dbl[])
        n125 = local read "ref mic wfm - dt"() -> (w258:dbl)
        n126 = local read "THD"() -> (w252:dbl[])
        n127 = local read "wfm - data"() -> (w255:dbl[])
        n128 = local read "wfm - dt"() -> (w256:dbl)
        n129 = Bundle("frequency (Hz)"=w254, "amplitude (dBr)"=w253) -> (w250:T11)  [unwired: 1 in]
        n130 = Bundle("frequency (Hz)"=w254, "THD"=w252) -> (w249:cluster{"frequency (Hz)":dbl[], "THD":dbl[]})  [unwired: 1 in]
        n131 = Bundle("frequency (Hz)"=w254, "THD+N"=w251) -> (w248:cluster{"frequency (Hz)":dbl[], "THD+N":dbl[]})  [unwired: 1 in]
        n132 = Bundle By Name("dt"=w256, "Y"=w255) -> (w261:waveform(dbl))  [unwired: 1 in]
        n133 = Bundle By Name("dt"=w258, "Y"=w257) -> (w260:waveform(dbl))  [unwired: 1 in]
        n134 = Build Array(w261, w260) -> (→"Time domain graph":waveform(dbl)[])
        n135 = Build Array(w250, w249, w248) -> (→"Sweep graph":cluster{"frequency (Hz)":dbl[], "THD+N":dbl[]}[])
      }
      frame "Update Sweep Graph Labels" {
        n136 = Unbundle By Name(w270) -> ("Visible Plot Id"=w267:i32)
        n137 = Type Cast(type=Y_axis_data_selection."Amplitude (dBr)" ("y-axis data"), x=w267) -> (*(type *) &x=w265:T8)
        n138 = Format Into String(format string="%s", w265) -> (resulting string=w264:string)  [unwired: 2 in, 1 out]
        n139 = control-ref of="Sweep graph"() -> (w269:refnum<vi>)
        n140 = property class="XYGraph (strict)"(reference=w269, "YScale.NameLbl.Text"=w264) -> ()  [unwired: 1 in, 2 out]
      }
      frame "Exit" {
        # "This case is triggered to close the User Interface from framework"
        n141 = Flush Queue(queue=w277, error in (no error)=w279) -> (queue out=w276:refnum<queue>, error out=w275:errorcluster)  [unwired: 1 out]
        n142 = Release Queue(queue=w276, force destroy? (F)=TRUE, error in (no error)=w275) -> (error out=w274:errorcluster)  [unwired: 2 out]
      }
      frame "Handle Error" {
      }
    }
  }
